vi "Hide Popup Image Window.vi"(8 "error in (no error)":errorcluster, 11 "UI in":refnum<class "UI.lvclass">) -> (0 "error out":errorcluster)   [LabVIEW 2020, in "AR Example.lvlib" / "UI.lvclass"]
uses:
  UI.lvclass
  Popup Image Window Action.ctl
  UI.lvclass/UI.ctl
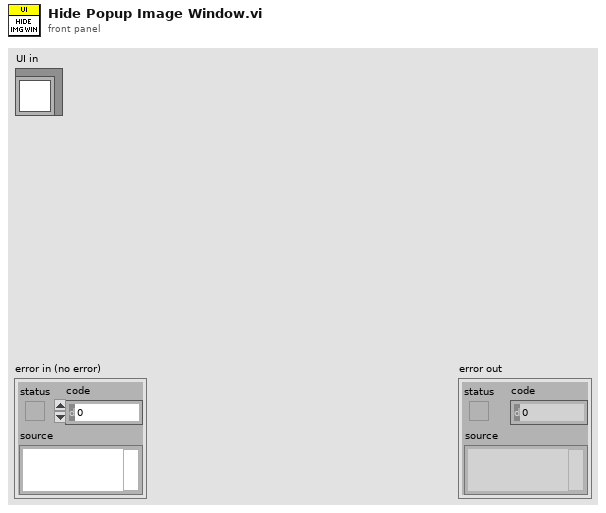
[diagram p1: front panel]
types:
  T1 = typedef "AR Example.lvlib/UI.lvclass/Popup Image Window Action.ctl" = enum16{"Show Panel", "Hide Panel", "Exit"}
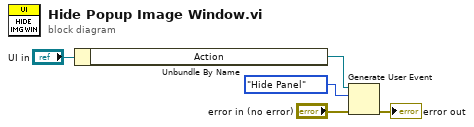
[diagram p0: block diagram]
diagram:
  n1 = Unbundle By Name("UI in") -> ("Action"=w4:refnum<user-event>)
  n2 = Generate User Event(user event=w4, event data cluster=Popup_Image_Window_Action."Hide Panel" ("event data"), error in="error in (no error)") -> (error out=→"error out":errorcluster)  [unwired: 1 in, 1 out]
